vi "add scan temp(SubVI).vi"(10 "字符串":string) -> (0 "布尔 3":bool, 2 "连接的字符串":string)   [LabVIEW 2019, in "SubVI.lvlib"]
uses:
  SubVI.lvlib
panel:
  in  "Number of Step":i32=10
  in  "Step Delay(secs)":dbl
  in  "Approach":i32(ring)=1 items=["FastSettle", "NoOvershoot", "Sweep"]
  in  "Increments(K)":dbl=10.0
  in  "cancel":bool
  in  "ok":bool
  in  "Rate(K/min)":dbl=10.0 min=0.0 max=10.0
  in  "Final Temp(K)":dbl=300.0 min=2.0 max=400.0
  in  "Initial Temp(K)":dbl=300.0 min=2.0 max=400.0
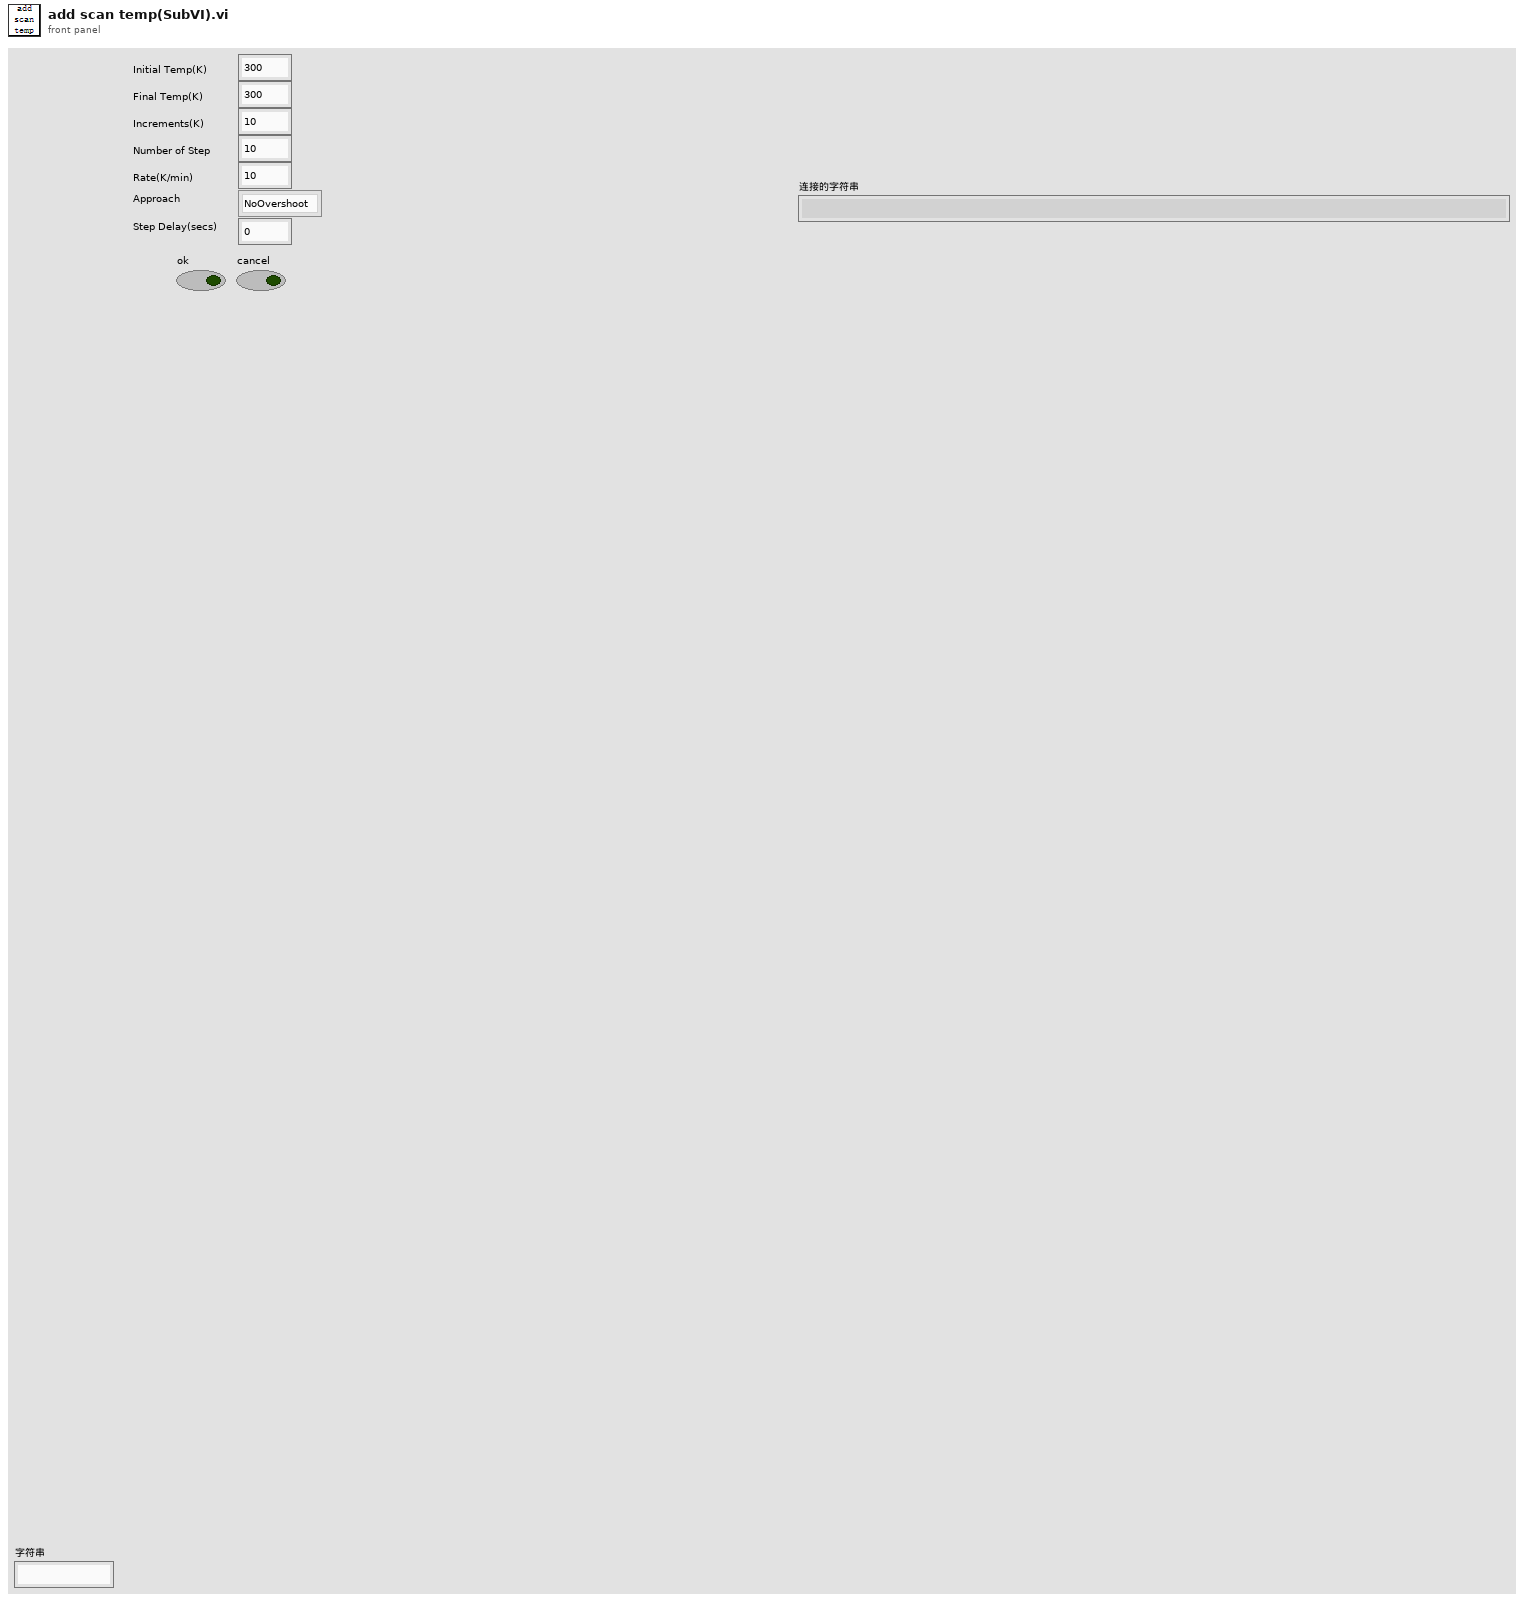
[diagram p1: front panel]
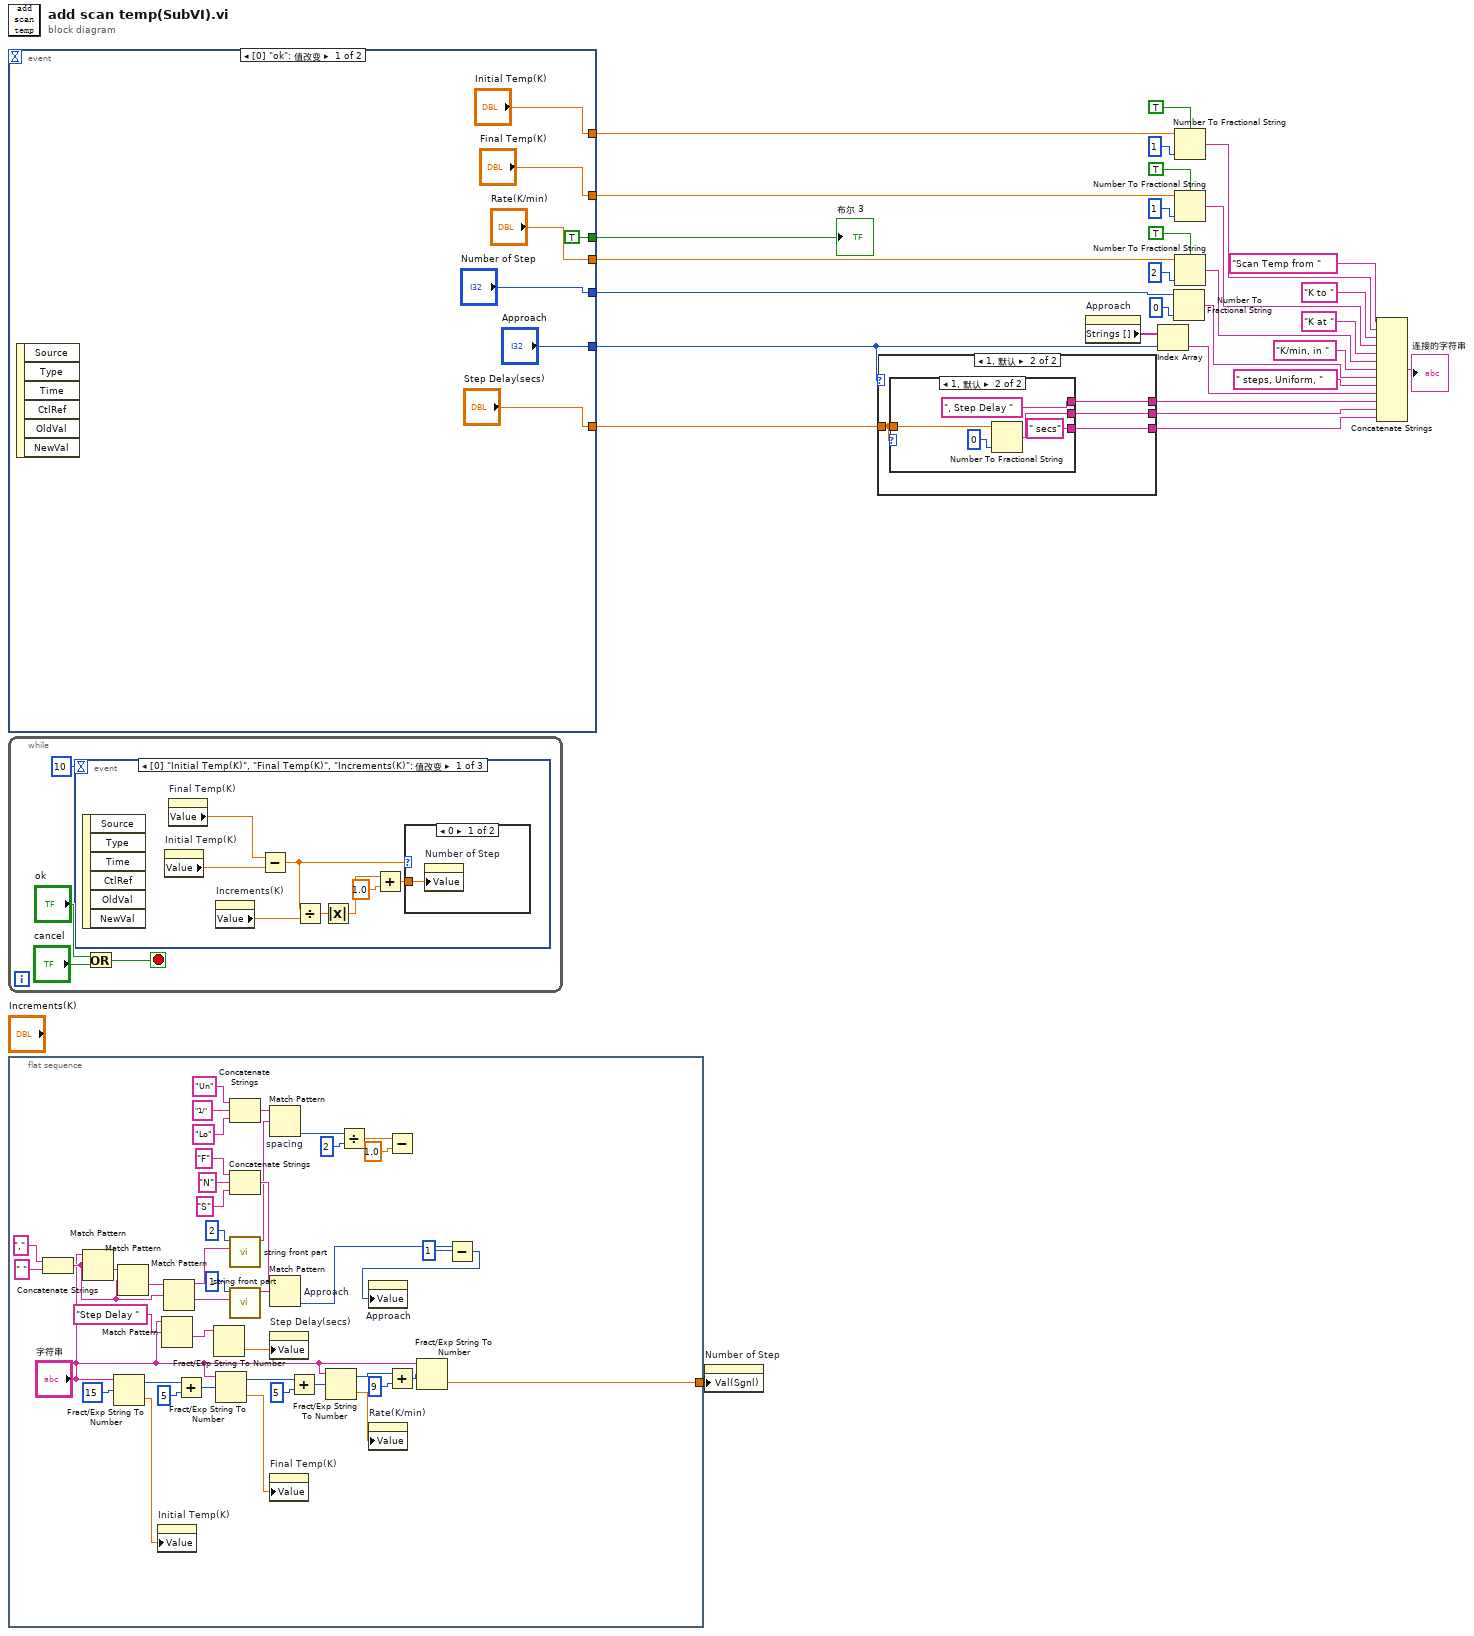
[diagram p0: block diagram]
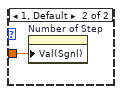
[diagram p2: hidden frame]
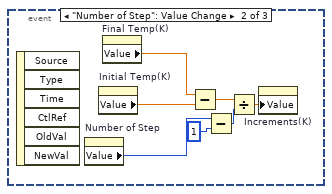
[diagram p3: hidden frame]
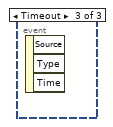
[diagram p4: hidden frame]
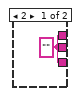
[diagram p5: hidden frame]
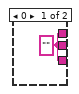
[diagram p6: hidden frame]
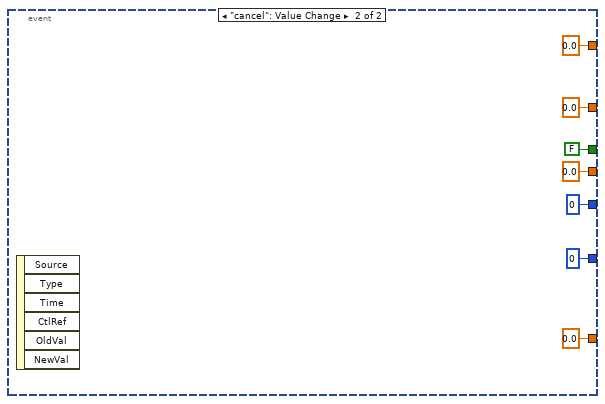
[diagram p7: hidden frame]
diagram:
  n1 = event shown="[0] \"ok\": 值改变" {
    selector: _ -> [_ _]
    dyn-events: _ -> [_ _]
    timeout: _ -> [_ _]
    tunnel: ["Final Temp(K)" 0.0 ("Field 2")] -> w19
    tunnel: ["Rate(K/min)" 0.0 ("Rate输入")] -> w16
    tunnel: ["Initial Temp(K)" 0.0 ("Field")] -> w28
    tunnel: [TRUE FALSE] -> w30
    tunnel: ["Number of Step" 0 ("Number of Step")] -> w13
    tunnel: ["Approach" 0 ("Approach输入")] -> w5
    tunnel: ["Step Delay(secs)" 0.0 ("Step Delay(secs)")] -> w6
    event "ok": Value Change {
      n2 = event-data() -> ()  [unwired: 1 in, 6 out]
    }
    event "cancel": Value Change {
      n3 = event-data() -> ()  [unwired: 1 in, 6 out]
    }
  }
  "布尔 3" <- w30
  n4 = while {
    stop <- w45 stop-if-true
    n5 = event shown="[0] \"Initial Temp(K)\", \"Final Temp(K)\", \"Increments(K)\": 值改变" {
      selector: _ -> [_ _ _]
      dyn-events: _ -> [_ _ _]
      timeout: 10 -> [_ _ _]
      event "Initial Temp(K)", "Final Temp(K)", "Increments(K)": Value Change {
        n6 = event-data() -> ()  [unwired: 1 in, 6 out]
        n7 = property on="Initial Temp(K)" class="DigNum (严格)"() -> ("Value"=w56:dbl)  [unwired: 2 in, 2 out]
        n8 = property on="Final Temp(K)" class="DigNum (严格)"() -> ("Value"=w51:dbl)  [unwired: 2 in, 2 out]
        n9 = property on="Increments(K)" class="DigNum (严格)"() -> ("Value"=w55:dbl)  [unwired: 2 in, 2 out]
        n10 = Subtract(x=w51, y=w56) -> (x-y=w50:dbl)
        n11 = Divide(x=w50, y=w55) -> (x/y=w53:dbl)
        n12 = Absolute Value(x=w53) -> (abs(x)=w52:dbl)
        n13 = Add(x=w52, y=1.0) -> (x+y=w49:dbl)
        n14 = case shown="0" w50 {
          tunnel: w49 -> [w57 w58]
          frame 0 {
            n15 = property on="Number of Step" class="DigNum (严格)"("Value"=w57) -> ()  [unwired: 2 in, 2 out]
          }
          frame 1, Default {
            n16 = property on="Number of Step" class="DigNum (严格)"("Val(Sgnl)"=w58) -> ()  [unwired: 2 in, 2 out]
          }
        }
      }
      event "Number of Step": Value Change {
        n17 = event-data() -> ()  [unwired: 1 in, 6 out]
        n18 = property on="Number of Step" class="DigNum (严格)"() -> ("Value"=w62:i32)  [unwired: 2 in, 2 out]
        n19 = property on="Initial Temp(K)" class="DigNum (严格)"() -> ("Value"=w64:dbl)  [unwired: 2 in, 2 out]
        n20 = property on="Final Temp(K)" class="DigNum (严格)"() -> ("Value"=w65:dbl)  [unwired: 2 in, 2 out]
        n21 = Subtract(x=w65, y=w64) -> (x-y=w63:dbl)
        n22 = Subtract(x=w62, y=1) -> (x-y=w60:i32)
        n23 = Divide(x=w63, y=w60) -> (x/y=w59:dbl)
        n24 = property on="Increments(K)" class="DigNum (严格)"("Value"=w59) -> ()  [unwired: 2 in, 2 out]
      }
      event Timeout {
        n25 = event-data() -> ()  [unwired: 1 in, 3 out]
      }
    }
    n26 = Or(x="ok", y="cancel") -> (x .or. y?=w45:bool)
  }
  n27 = flat-sequence {
    tunnel: [w73] -> w1
    frame #0 {
      n28 = Concatenate Strings("," ("字符串"), " " ("字符串")) -> (w91:string)
      n29 = Match Pattern(string="字符串", regular expression=w91) -> (after substring=w109:string)  [unwired: 1 in, 3 out]
      n30 = Fract/Exp String To Number(string="字符串", offset=15 ("偏移量")) -> (offset past number=w107:i32, number=w71:dbl)  [unwired: 2 in]
      n31 = Match Pattern(string=w109, regular expression=w91) -> (after substring=w92:string)  [unwired: 1 in, 3 out]
      n32 = property on="Initial Temp(K)" class="DigNum (严格)"("Value"=w71) -> ()  [unwired: 2 in, 2 out]
      n33 = Match Pattern(string="字符串", regular expression="Step Delay ") -> (after substring=w76:string)  [unwired: 1 in, 3 out]
      n34 = Match Pattern(string=w92, regular expression=w91) -> (before substring=w90:string, after substring=w78:string)  [unwired: 1 in, 2 out]
      n35 = Add(x=w107, y=5) -> (x+y=w106:i32)
      n36 = Fract/Exp String To Number(string=w76) -> (number=w72:dbl)  [unwired: 3 in, 1 out]
      n37 = Fract/Exp String To Number(string="字符串", offset=w106) -> (offset past number=w97:i32, number=w69:dbl)  [unwired: 2 in]
      n38 = Concatenate Strings("Un" ("字符串"), "1/" ("字符串"), "Lo" ("字符串")) -> (w84:string)
      n39 = Concatenate Strings("F" ("字符串"), "N" ("字符串"), "S" ("字符串")) -> (w100:string)
      n40 = call "string front part.vi"("字符串"=w90, "偏移量(0)"=2) -> ("result string"=w88:string)  [unwired: 9 in]
      n41 = call "string front part.vi"("字符串"=w78, "偏移量(0)"=1) -> ("result string"=w103:string)  [unwired: 9 in]
      n42 = Match Pattern "spacing"(string=w84, regular expression=w88) -> (offset past match=w83:i32)  [unwired: 1 in, 3 out]
      n43 = Match Pattern "Approach"(string=w100, regular expression=w103) -> (offset past match=w68:i32)  [unwired: 1 in, 3 out]
      n44 = property on="Step Delay(secs)" class="DigNum (严格)"("Value"=w72) -> ()  [unwired: 2 in, 2 out]
      n45 = property on="Final Temp(K)" class="DigNum (严格)"("Value"=w69) -> ()  [unwired: 2 in, 2 out]
      n46 = Add(x=w97, y=5) -> (x+y=w95:i32)
      n47 = Fract/Exp String To Number(string="字符串", offset=w95) -> (offset past number=w79:i32, number=w70:dbl)  [unwired: 2 in]
      n48 = Divide(x=w83, y=2) -> (x/y=w81:dbl)
      n49 = property on="Rate(K/min)" class="DigNum (严格)"("Value"=w70) -> ()  [unwired: 2 in, 2 out]
      n50 = Subtract(x=w81, y=1.0) -> ()  [unwired: 1 out]
      n51 = Add(x=w79, y=9) -> (x+y=w93:i32)
      n52 = Fract/Exp String To Number(string="字符串", offset=w93) -> (number=w73:dbl)  [unwired: 2 in, 1 out]
      n53 = Subtract(x=w68, y=1) -> (x-y=w66:i32)
      n54 = property on="Approach" class="Ring (严格)"("Value"=w66) -> ()  [unwired: 2 in, 2 out]
    }
  }
  n55 = property on="Number of Step" class="DigNum (严格)"("Val(Sgnl)"=w1) -> ()  [unwired: 2 in, 2 out]
  n56 = case shown="1, 默认" w5 {
    tunnel: [w110 w114] -> w4
    tunnel: [w110 w113] -> w2
    tunnel: w6 -> [_ w111]
    tunnel: [w110 w112] -> w3
    frame 2 {
      w110 = ""
    }
    frame 1, Default {
      n57 = case shown="1, 默认" w111 {
        tunnel: [w115 ", Step Delay " ("字符串")] -> w114
        tunnel: [w115 " secs" ("字符串")] -> w113
        tunnel: w111 -> [_ w118]
        tunnel: [w115 w117] -> w112
        frame 0 {
          w115 = ""
        }
        frame 1, Default {
          n58 = Number To Fractional String(number=w118, precision (6)=i16 0 ("精度(6)")) -> (F-format string=w117:string)  [unwired: 2 in]
        }
      }
    }
  }
  n59 = property on="Approach" class="Ring (严格)"() -> ("Strings []"=w7:string[])  [unwired: 2 in, 2 out]
  n60 = Index Array(array=w7, index=w5) -> (element=w9:string)
  n61 = Number To Fractional String(number=w13, precision (6)=i16 0 ("精度(6)")) -> (F-format string=w12:string)  [unwired: 2 in]
  n62 = Number To Fractional String(use system decimal point (T)=TRUE ("使用系统小数点(T)"), number=w28, precision (6)=i16 1 ("精度(6)")) -> (F-format string=w26:string)  [unwired: 1 in]
  n63 = Number To Fractional String(use system decimal point (T)=TRUE ("使用系统小数点(T)"), number=w19, precision (6)=i16 1 ("精度(6)")) -> (F-format string=w21:string)  [unwired: 1 in]
  n64 = Number To Fractional String(use system decimal point (T)=TRUE ("使用系统小数点(T)"), number=w16, precision (6)=i16 2 ("精度(6)")) -> (F-format string=w15:string)  [unwired: 1 in]
  n65 = Concatenate Strings("Scan Temp from " ("字符串"), w26, "K to " ("字符串"), w21, "K at " ("字符串"), w15, "K/min, in " ("字符串"), w12, " steps, Uniform, " ("字符串"), w9, w4, w3, w2) -> (→"连接的字符串":string)
